vi "motor_server.vi"(10 "motor load":bool, 11 "motor":refnum<visa-resource-name>="COM21") -> ()   [LabVIEW 2020]
uses:
  <vilib>/NI/Modbus Library/API/Wrapper/Create Serial Master.vi
  status/stop software.vi
  status/emergency stop.vi
  status/pause1.vi
  status/pause2.vi
  status/pause3.vi
  status/pause4.vi
  <vilib>/NI/Modbus Library/API/Master/Modbus Master.lvclass
  <vilib>/NI/Modbus Library/API/Wrapper/API Main.lvlib
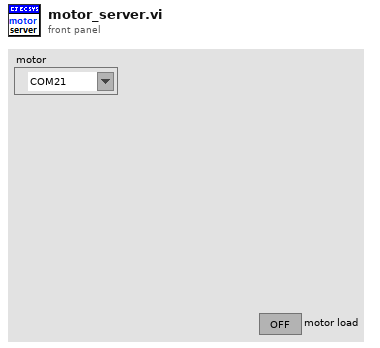
[diagram p1: front panel]
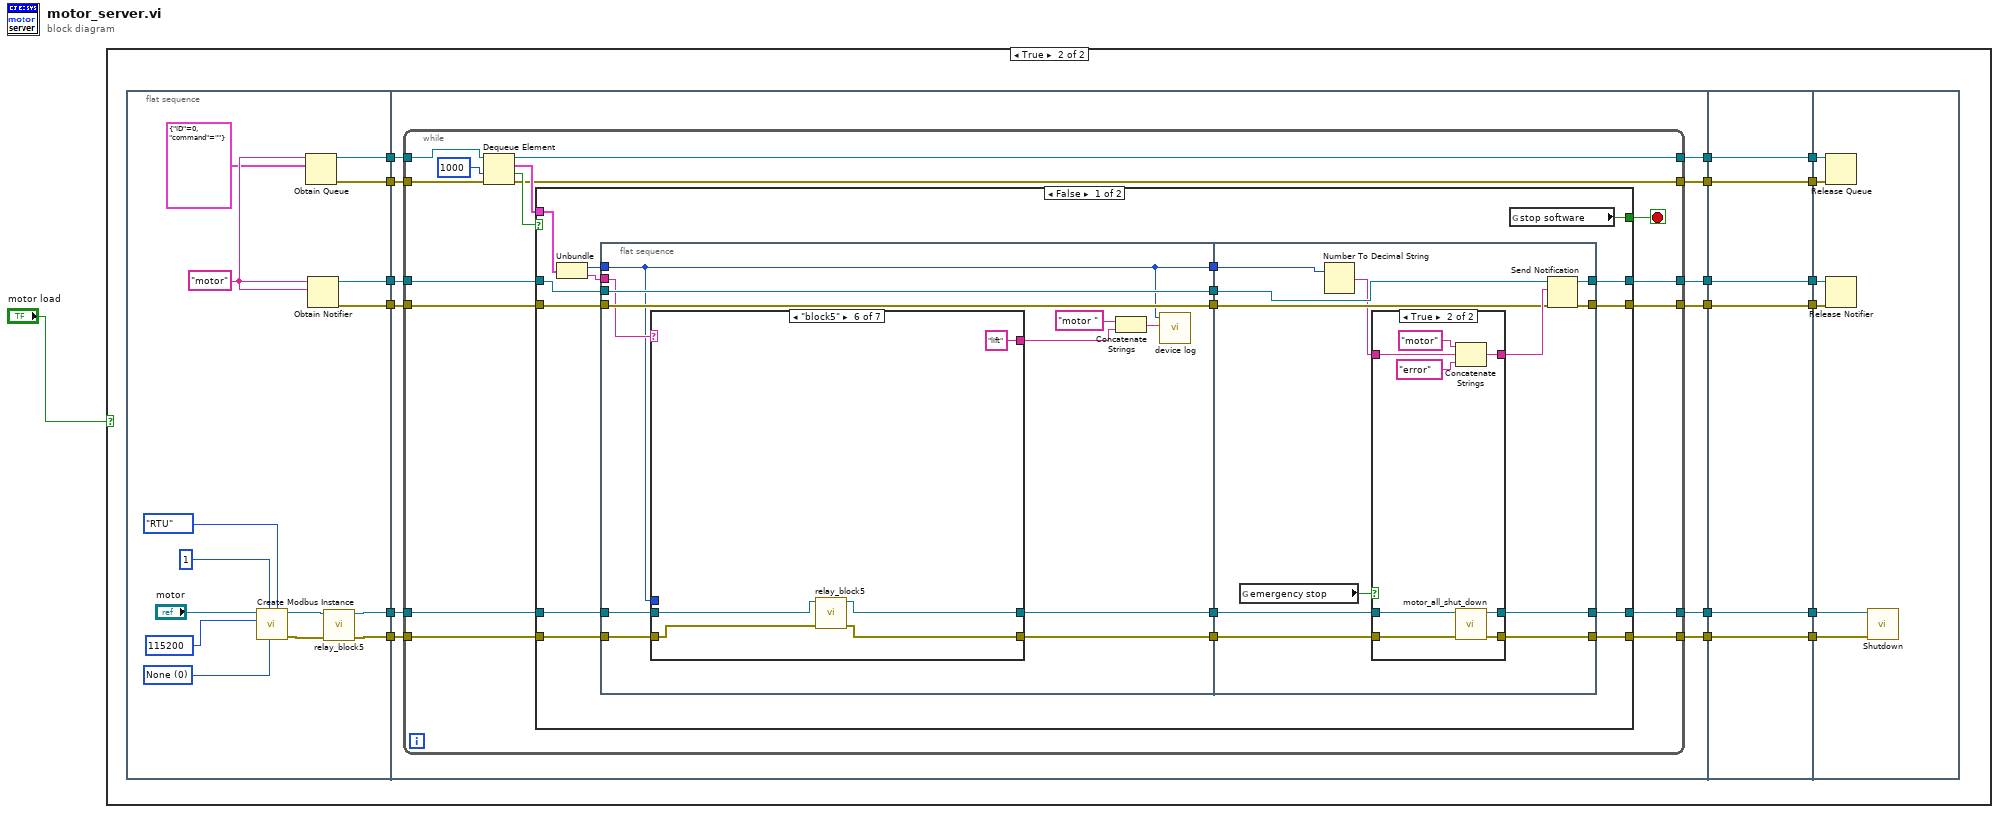
[diagram p0: block diagram]
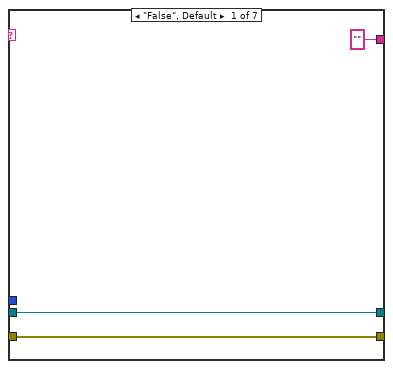
[diagram p3: hidden frame]
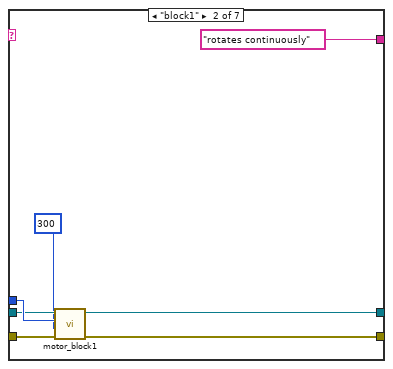
[diagram p4: hidden frame]
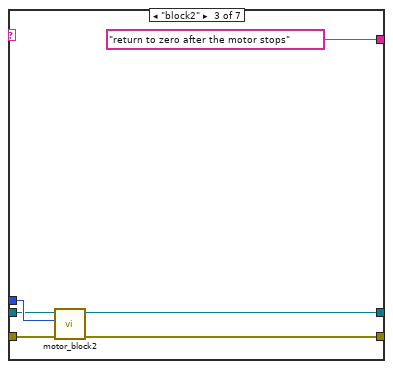
[diagram p5: hidden frame]
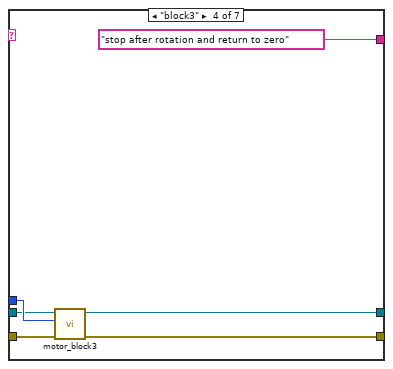
[diagram p6: hidden frame]
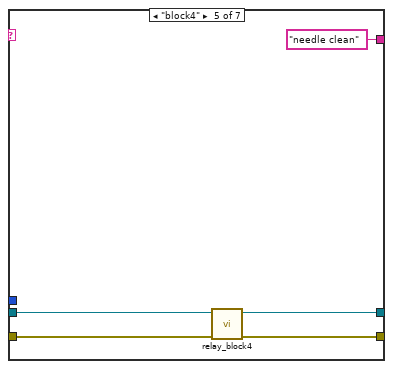
[diagram p7: hidden frame]
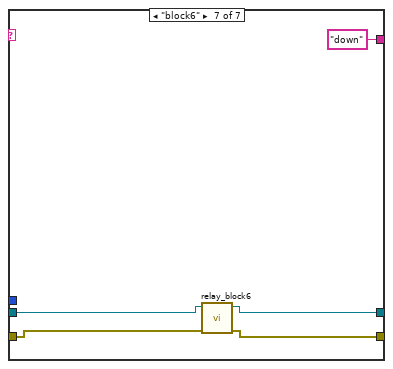
[diagram p8: hidden frame]
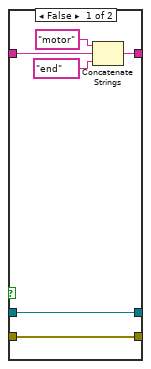
[diagram p9: hidden frame]
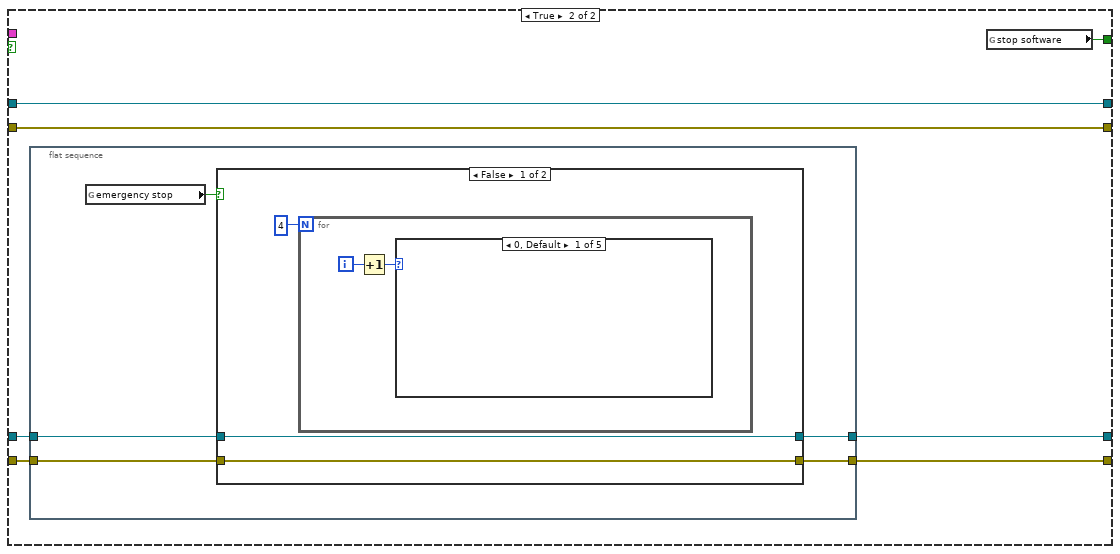
[diagram p10: hidden frame]
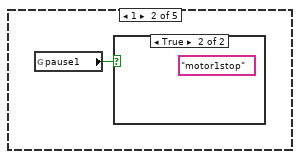
[diagram p11: hidden frame]
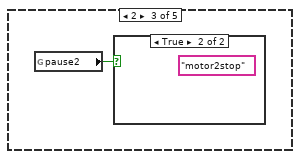
[diagram p13: hidden frame]
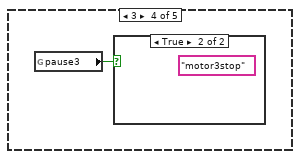
[diagram p15: hidden frame]
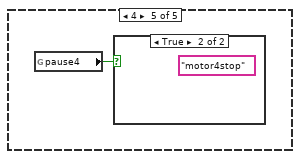
[diagram p17: hidden frame]
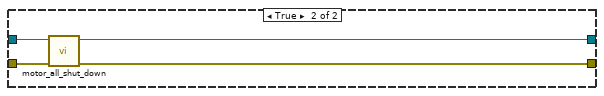
[diagram p19: hidden frame]
diagram:
  n1 = case shown="True" "motor load" {
    frame False {
    }
    frame True {
      n2 = flat-sequence {
        tunnel: [w34] -> w19
        tunnel: [w33] -> w18
        tunnel: [w32] -> w17
        tunnel: [w31] -> w16
        tunnel: [w23] -> w15
        tunnel: [w20] -> w14
        tunnel: w19 -> [w46]
        tunnel: w18 -> [w45]
        tunnel: w17 -> [w44]
        tunnel: w16 -> [w43]
        tunnel: [w42] -> w13
        tunnel: [w41] -> w12
        tunnel: [w40] -> w11
        tunnel: [w39] -> w10
        tunnel: w15 -> [w38]
        tunnel: w14 -> [w37]
        tunnel: [w36] -> w9
        tunnel: [w35] -> w8
        tunnel: w13 -> [w184]
        tunnel: [w184] -> w7
        tunnel: w12 -> [w183]
        tunnel: [w183] -> w6
        tunnel: w11 -> [w182]
        tunnel: [w182] -> w5
        tunnel: w10 -> [w181]
        tunnel: [w181] -> w4
        tunnel: w9 -> [w180]
        tunnel: [w180] -> w3
        tunnel: w8 -> [w179]
        tunnel: [w179] -> w2
        tunnel: w7 -> [w190]
        tunnel: w6 -> [w189]
        tunnel: w5 -> [w188]
        tunnel: w4 -> [w187]
        tunnel: w3 -> [w185]
        tunnel: w2 -> [w186]
        frame #0 {
          w26 = u16 0 items=["None", "Odd", "Even", "Mark", "Space"] ("parity (even)")
          w30 = "motor" ("name (unnamed)")
          n3 = call-poly <vilib>:"Create Modbus Instance.vi"("serial type"=enum16{"RTU", "ASCII"}."RTU", "parity (even)"=w26, "unit ID"=u8 1, "baud rate"=u32 115200, "VISA resource name"="motor") -> ("error out"=w21:errorcluster, "serial master instance"=w22:refnum<class "Modbus Master.lvclass">)  [unwired: 5 in]
          n4 = Obtain Queue(name (unnamed)=w30, element data type=cluster{"ID":i32, "command":string} {"ID"=0, "command"=""} ("参数")) -> (queue out=w34:refnum<queue>, error out=w33:errorcluster)  [unwired: 3 in, 1 out]
          n5 = Obtain Notifier(name (unnamed)=w30, notification data type=w30) -> (notifier out=w32:refnum<notifier>, error out=w31:errorcluster)  [unwired: 2 in, 1 out]
          n6 = call "relay_block5.vi"("error in"=w21, "Modbus master in"=w22) -> ("error out"=w20:errorcluster, "Modbus master out"=w23:refnum<class "Modbus Master.lvclass">)  [unwired: 8 in]
        }
        frame #1 {
          n7 = while {
            tunnel: w46 -> [w61]
            tunnel: w45 -> [w60]
            tunnel: w44 -> [w56]
            tunnel: w43 -> [w55]
            tunnel: [w54] -> w42
            tunnel: [w53] -> w41
            tunnel: [w52] -> w40
            tunnel: [w51] -> w39
            tunnel: w38 -> [w50]
            tunnel: w37 -> [w49]
            tunnel: [w48] -> w36
            tunnel: [w47] -> w35
            stop <- w58 stop-if-true
            n8 = Dequeue Element(queue=w61, timeout in ms (-1)=1000, error in (no error)=w60) -> (queue out=w52:refnum<queue>, element=w57:cluster{"ID":i32, "command":string}, timed out?=w59:bool, error out=w51:errorcluster)
            n9 = case shown="False" w59 {
              tunnel: [w71 w158] -> w58
              tunnel: w57 -> [w79 _]
              tunnel: w56 -> [w78 w160]
              tunnel: w55 -> [w73 w159]
              tunnel: [w76 w160] -> w54
              tunnel: [w75 w159] -> w53
              tunnel: w50 -> [w70 w157]
              tunnel: w49 -> [w69 w156]
              tunnel: [w66 w155] -> w48
              tunnel: [w65 w154] -> w47
              frame False {
                n10 = Unbundle(w79) -> ("ID"=w64:i32, "command"=w74:string)
                n11 = flat-sequence {
                  tunnel: w64 -> [w81]
                  tunnel: w78 -> [w90]
                  tunnel: [w90] -> w77
                  tunnel: w74 -> [w88]
                  tunnel: w73 -> [w89]
                  tunnel: [w89] -> w72
                  tunnel: w70 -> [w86]
                  tunnel: w69 -> [w85]
                  tunnel: [w84] -> w68
                  tunnel: [w83] -> w67
                  tunnel: [w81] -> w63
                  tunnel: [w138] -> w76
                  tunnel: [w137] -> w75
                  tunnel: w77 -> [w136]
                  tunnel: w72 -> [w135]
                  tunnel: w68 -> [w133]
                  tunnel: w67 -> [w132]
                  tunnel: [w131] -> w66
                  tunnel: [w130] -> w65
                  tunnel: w63 -> [w128]
                  frame #0 {
                    n12 = case shown="\"block5\"" w88 {
                      tunnel: [w92 w95 w101 w107 w117 w120 w125] -> w84
                      tunnel: w86 -> [w92 w97 w103 w109 w115 w122 w127]
                      tunnel: w85 -> [w91 w99 w105 w111 w114 w121 w126]
                      tunnel: w81 -> [_ w98 w104 w110 _ _ _]
                      tunnel: [w91 w96 w102 w108 w116 w119 w124] -> w83
                      tunnel: ["" ("String") "rotates continuously" ("string") "return to zero after the motor stops" ("string") "stop after rotation and return to zero" ("string") "needle clean" ("string") "lift" ("string") "down" ("string")] -> w80
                      frame "False", Default {
                      }
                      frame "block1" {
                        n13 = call "motor_block1.vi"("error in"=w99, "rotate rate"=u16 300, "unit ID"=w98, "Modbus master in"=w97) -> ("error out"=w96:errorcluster, "Modbus master out"=w95:refnum<class "Modbus Master.lvclass">)  [unwired: 6 in]
                      }
                      frame "block2" {
                        n14 = call "motor_block2.vi"("error in"=w105, "unit ID"=w104, "Modbus master in"=w103) -> ("error out"=w102:errorcluster, "Modbus master out"=w101:refnum<class "Modbus Master.lvclass">)  [unwired: 7 in]
                      }
                      frame "block3" {
                        n15 = call "motor_block3.vi"("error in"=w111, "unit ID"=w110, "Modbus master in"=w109) -> ("error out"=w108:errorcluster, "Modbus master out"=w107:refnum<class "Modbus Master.lvclass">)  [unwired: 7 in]
                      }
                      frame "block4" {
                        n16 = call "relay_block4.vi"("error in"=w114, "Modbus master in"=w115) -> ("error out"=w116:errorcluster, "Modbus master out"=w117:refnum<class "Modbus Master.lvclass">)  [unwired: 8 in]
                      }
                      frame "block5" {
                        n17 = call "relay_block5.vi"("error in"=w121, "Modbus master in"=w122) -> ("error out"=w119:errorcluster, "Modbus master out"=w120:refnum<class "Modbus Master.lvclass">)  [unwired: 8 in]
                      }
                      frame "block6" {
                        n18 = call "relay_block6.vi"("error in"=w126, "Modbus master in"=w127) -> ("error out"=w124:errorcluster, "Modbus master out"=w125:refnum<class "Modbus Master.lvclass">)  [unwired: 8 in]
                      }
                    }
                    n19 = Concatenate Strings("motor " ("string"), w80) -> (w82:string)
                    n20 = call "device log.vi"("new element/subarray"=w82, "worker ID"=w81) -> ()  [unwired: 10 in]
                  }
                  frame #1 {
                    n21 = global read "emergency stop.vi" "emergency stop"() -> (w134:bool)
                    n22 = Number To Decimal String(number=w128) -> (decimal integer string=w129:string)  [unwired: 1 in]
                    n23 = case shown="True" w134 {
                      tunnel: [w142 w151] -> w139
                      tunnel: w129 -> [w143 w150]
                      tunnel: w133 -> [w141 w148]
                      tunnel: w132 -> [w140 w149]
                      tunnel: [w141 w146] -> w131
                      tunnel: [w140 w147] -> w130
                      frame False {
                        n24 = Concatenate Strings("motor" ("string"), w143, "end" ("notification")) -> (w142:string)
                      }
                      frame True {
                        n25 = Concatenate Strings("motor" ("string"), w150, "error" ("notification")) -> (w151:string)
                        n26 = call "motor_all_shut_down.vi"("error in"=w149, "Modbus master in"=w148) -> ("error out"=w147:errorcluster, "Modbus master out"=w146:refnum<class "Modbus Master.lvclass">)  [unwired: 8 in]
                      }
                    }
                    n27 = Send Notification(notification=w139, notifier=w136, error in (no error)=w135) -> (notifier out=w138:refnum<notifier>, error out=w137:errorcluster)
                  }
                }
                n28 = global read "stop software.vi" "stop software"() -> (w71:bool)
              }
              frame True {
                n29 = flat-sequence {
                  tunnel: w157 -> [w164]
                  tunnel: w156 -> [w163]
                  tunnel: [w162] -> w155
                  tunnel: [w161] -> w154
                  frame #0 {
                    n30 = global read "emergency stop.vi" "emergency stop"() -> (w165:bool)
                    n31 = case shown="False" w165 {
                      tunnel: w164 -> [w167 w178]
                      tunnel: w163 -> [w166 w177]
                      tunnel: [w167 w176] -> w162
                      tunnel: [w166 w175] -> w161
                      frame False {
                        n32 = for {
                          N: 4 -> [_]
                          i -> [w170]
                          n33 = Increment(x=w170) -> (x+1=w169:i32)
                          n34 = case shown="0, Default" w169 {
                            frame 0, Default {
                            }
                            frame 1 {
                              n35 = global read "pause1.vi" "pause1"() -> (w171:bool)
                              n36 = case shown="True" w171 {
                                frame False {
                                }
                                frame True {
                                (unwired) "motor1stop" ("motor status")
                                }
                              }
                            }
                            frame 2 {
                              n37 = global read "pause2.vi" "pause2"() -> (w172:bool)
                              n38 = case shown="True" w172 {
                                frame False {
                                }
                                frame True {
                                (unwired) "motor2stop" ("motor status")
                                }
                              }
                            }
                            frame 3 {
                              n39 = global read "pause3.vi" "pause3"() -> (w173:bool)
                              n40 = case shown="True" w173 {
                                frame False {
                                }
                                frame True {
                                (unwired) "motor3stop" ("motor status")
                                }
                              }
                            }
                            frame 4 {
                              n41 = global read "pause4.vi" "pause4"() -> (w174:bool)
                              n42 = case shown="True" w174 {
                                frame False {
                                }
                                frame True {
                                (unwired) "motor4stop" ("motor status")
                                }
                              }
                            }
                          }
                        }
                      }
                      frame True {
                        n43 = call "motor_all_shut_down.vi"("error in"=w177, "Modbus master in"=w178) -> ("error out"=w175:errorcluster, "Modbus master out"=w176:refnum<class "Modbus Master.lvclass">)  [unwired: 8 in]
                      }
                    }
                  }
                }
                n44 = global read "stop software.vi" "stop software"() -> (w158:bool)
              }
            }
          }
        }
        frame #2 {
        }
        frame #3 {
          n45 = Release Queue(queue=w188, error in (no error)=w187) -> ()  [unwired: 1 in, 3 out]
          n46 = Release Notifier(notifier=w190, error in (no error)=w189) -> ()  [unwired: 1 in, 3 out]
          n47 = call-dynamic "Shutdown.vi"("error in"=w186, "Modbus master in"=w185) -> ()  [unwired: 9 in, 1 out]
        }
      }
    }
  }
